vi "ConvertTo(waveform).vi"(8 "error in":errorcluster, 9 "Message Payload":variant) -> (0 "error out":errorcluster, 1 "d Cmd Payload":T1)   [LabVIEW 2019]
doc: "Convert variant to DAQmx waveform type\n\nBolder Software LLC"
uses:
  Classes/Datalog/DatalogSubvis/SearchableTag.ctl
  Classes/Sequence/SequenceSubvis/RF Direction.ctl
  Classes/Sequence/SequenceSubvis/PolarizationSelect.ctl
  Classes/Datalog/DataLog.lvclass
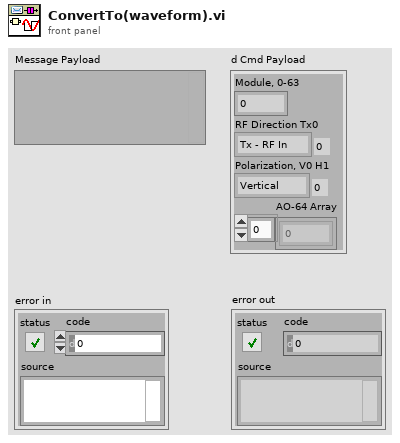
[diagram p1: front panel]
types:
  T1 = typedef "DataLog.lvclass/SearchableTag.ctl" = cluster{"Module, 0-63":i32, "RF Direction Tx0":T2, "Polarization, V0 H1":T3, "AO-64 Array":dbl[]}
  T2 = typedef "RF Direction.ctl" = enum16{"Tx - RF In", "Rx - RF Out"}
  T3 = typedef "PolarizationSelect.ctl" = enum16{"Vertical", "Horizontal"}
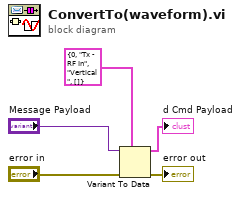
[diagram p0: block diagram]
diagram:
  n1 = Variant To Data(error in="error in", type=T1 {"Module, 0-63"=0, "RF Direction Tx0"=enum."Tx - RF In", "Polarization, V0 H1"=enum."Vertical", "AO-64 Array"=[]} ("d Cmd Payload"), Variant="Message Payload") -> (data=→"d Cmd Payload":T1, error out=→"error out":errorcluster)
